vi "Find Octave Executable Future Versions.vi"() -> (1 "Found executable?":bool, 3 "Executable path":path)   [LabVIEW 2020, in "GOLPI library.lvlib"]
doc: "Tries to find GNU Octave binary for future versions of GNU Octave at default installation paths."
uses:
  GOLPI library.lvlib
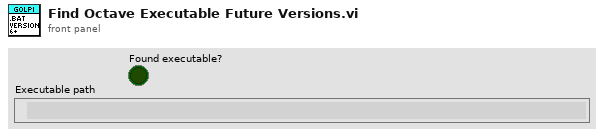
[diagram p1: front panel]
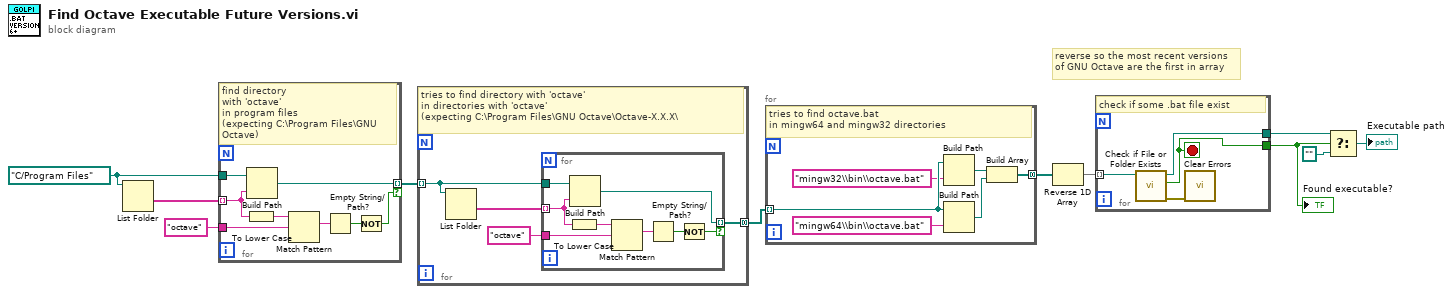
[diagram p0: block diagram]
diagram:
  w3 = path "C:/Program Files" ("path")
  # "reverse so the most recent versions\nof GNU Octave are the first in array"
  n1 = List Folder(path=w3) -> (folder names=w2:string[])  [unwired: 3 in, 3 out]
  n2 = for {
    tunnel: w2 -> [w17] mode=indexing
    tunnel: w3 -> [w18]
    tunnel: [w16] -> w5 mode=indexing if=w13
    tunnel: "octave" ("regular expression") -> [w12]
    # "find directory\nwith 'octave'\nin program files\n(expecting C:\\Program Files\\GNU Octave)"
    n3 = To Lower Case(string=w17) -> (all lower case string=w19:string)
    n4 = Build Path(base path=w18, name or relative path=w17) -> (appended path=w16:path)
    n5 = Match Pattern(string=w19, regular expression=w12) -> (match substring=w15:string)  [unwired: 1 in, 3 out]
    n6 = Empty String/Path?(string/path=w15) -> (empty?=w14:bool)
    n7 = Not(x=w14) -> (.not. x?=w13:bool)
  }
  n8 = for {
    tunnel: w5 -> [w22] mode=indexing
    tunnel: [w21] -> w6 mode=concatenating
    # "tries to find directory with 'octave'\nin directories with 'octave'\n(expecting C:\\Program Files\\GNU Octave\\Octave-X.X.X\\"
    n9 = List Folder(path=w22) -> (folder names=w23:string[])  [unwired: 3 in, 3 out]
    n10 = for {
      tunnel: w23 -> [w29] mode=indexing
      tunnel: w22 -> [w30]
      tunnel: [w28] -> w21 mode=indexing if=w25
      tunnel: "octave" ("regular expression") -> [w24]
      n11 = To Lower Case(string=w29) -> (all lower case string=w31:string)
      n12 = Build Path(base path=w30, name or relative path=w29) -> (appended path=w28:path)
      n13 = Match Pattern(string=w31, regular expression=w24) -> (match substring=w27:string)  [unwired: 1 in, 3 out]
      n14 = Empty String/Path?(string/path=w27) -> (empty?=w26:bool)
      n15 = Not(x=w26) -> (.not. x?=w25:bool)
    }
  }
  n16 = for {
    tunnel: w6 -> [w37] mode=indexing
    tunnel: [w33] -> w7 mode=concatenating
    # "tries to find octave.bat\nin mingw64 and mingw32 directories"
    n17 = Build Path(base path=w37, name or relative path="mingw32\\bin\\octave.bat" ("format string")) -> (appended path=w34:path)
    n18 = Build Path(base path=w37, name or relative path="mingw64\\bin\\octave.bat" ("format string")) -> (appended path=w35:path)
    n19 = Build Array(w34, w35) -> (w33:path[])
  }
  n20 = Reverse 1D Array(array=w7) -> (reversed array=w8:path[])
  n21 = for {
    tunnel: w8 -> [w41] mode=indexing
    tunnel: [w39] -> w10
    tunnel: [w38] -> w9
    stop <- w38 stop-if-true
    # "check if some .bat file exist"
    n22 = call <vilib>:"Check if File or Folder Exists.vi"("path"=w41) -> ("error out"=w40:errorcluster, "file or folder exists?"=w38:bool, "dup path"=w39:path)  [unwired: 8 in]
    n23 = call <vilib>:"Clear Errors.vi"("error in (no error)"=w40) -> ()  [unwired: 5 in, 2 out]
  }
  "Found executable?" <- w9
  n24 = Select(t=w10, s=w9, f=path "") -> (s? t:f=→"Executable path":path)
